vi "Oscilloscope_Interface.vi"() -> ()   [LabVIEW 2020]
uses:
  Tektronix 7000 Series/Library/Tektronix 7000 Series.lvlib
panel:
  out "Active_Channels":u16[](array[numeric])
  out "Get #Averages":i32
  in  "Go2":bool
  in  "Set Vertical Scale Button":bool
  in  "Channels Position":bool
  in  "Channels Bandwidth":bool
  in  "Default Setup Button":bool
  in  "Set Mode":bool
  in  "Autosetup":bool
  out "Oscilloscope Mode":string
  out "Synch Variable":bool
  out "S4":bool
  out "S3":bool
  out "S2":bool
  out "S1":bool
  out "Acquisition":bool
  in  "Configure Digital Channel":bool
  in  "Configure Measurement":bool
  in  "Configure Acquisition":bool
  in  "Timebase Configuration":bool
  in  "Cursor Configuration":bool
  in  "Histogram Configuration":bool
  in  "Set Horizontal Scale Button":bool
  in  "Go1":bool
  out "Measurement":dbl
  in  "Select a Channel for the Operation":i8(knob) scale=1.0..4.0
  in  "Trigger Configuration":bool
  in  "FunctionA":u16(ring) items=["Amplitude", "RMS", "Pk-Pk", "High", "Max", "Cycle RMS", "Low", "Min", "+Ovt shoot", "-Ovt shoot", "Cycle Mean", "Mean"]
  in  "Channels Configuration":bool
  out "Go!":bool
  out "Error!":bool
  in  "Synchronization":bool
  out "Display Message":string
  out "End Variable":bool
  out "Save Variable":bool
  in  "Operating Modes":bool
  in  "Pause Button":bool
  in  "Play Button":bool
  in  "End Button":bool
  in  "Guide Button":bool
  in  "Save Button":bool
  in  "Ch 4":bool
  in  "Ch 3":bool
  in  "Ch 2":bool
  in  "Ch 1":bool
  out "Running?":bool
  in  "Set Oscilloscope Mode":u16(ring) items=["Continuous", "Single"]
  in  "Set Sampling Mode":bool
  in  "Set Acquisition Mode":bool
  in  "Set Number of Averages":bool
  out "Master?":bool
  in  "Set Acquisition Mode":u16(ring) items=["Sample", "Peak Detect", "High resolution", "Average", "WFMDB", "Envelope"]
  out "Tektronix 7000 Oscilloscope":waveform(dbl)[](graph) caption="Oscilloscope"
  in  "Set Sampling Mode":u16(ring) items=["Real Time", "Equivalent Time", "Interpolation"]
  in  "Set #Averages":i32
  # "Tektronix DPO75002SX ATI Performance              Andrea Perna's Thesis"
  # "Channels Activation"
  # "Variables"
  # "Function"
  # "Set #Averages"
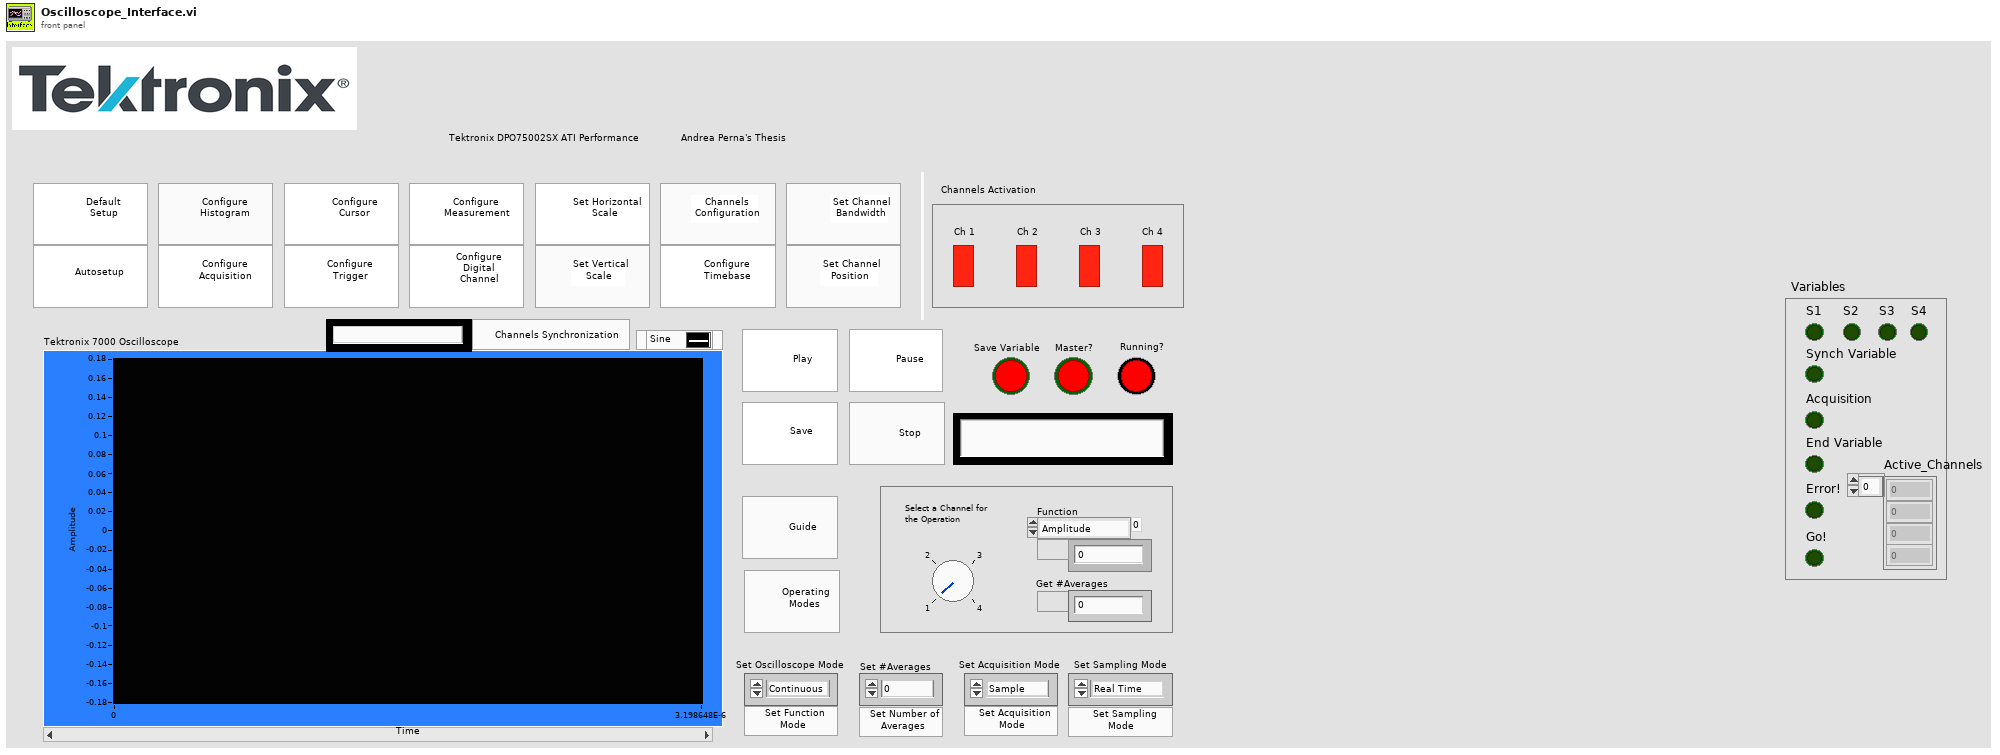
[diagram p1: front panel]
types:
  T1 = enum8{"Enabled", "Disabled", "Disabled and Grayed Out"}
  T2 = cluster{"Parameters(array)":string[], "Waveform Data":waveform(dbl)[], "array":u16[], bool}
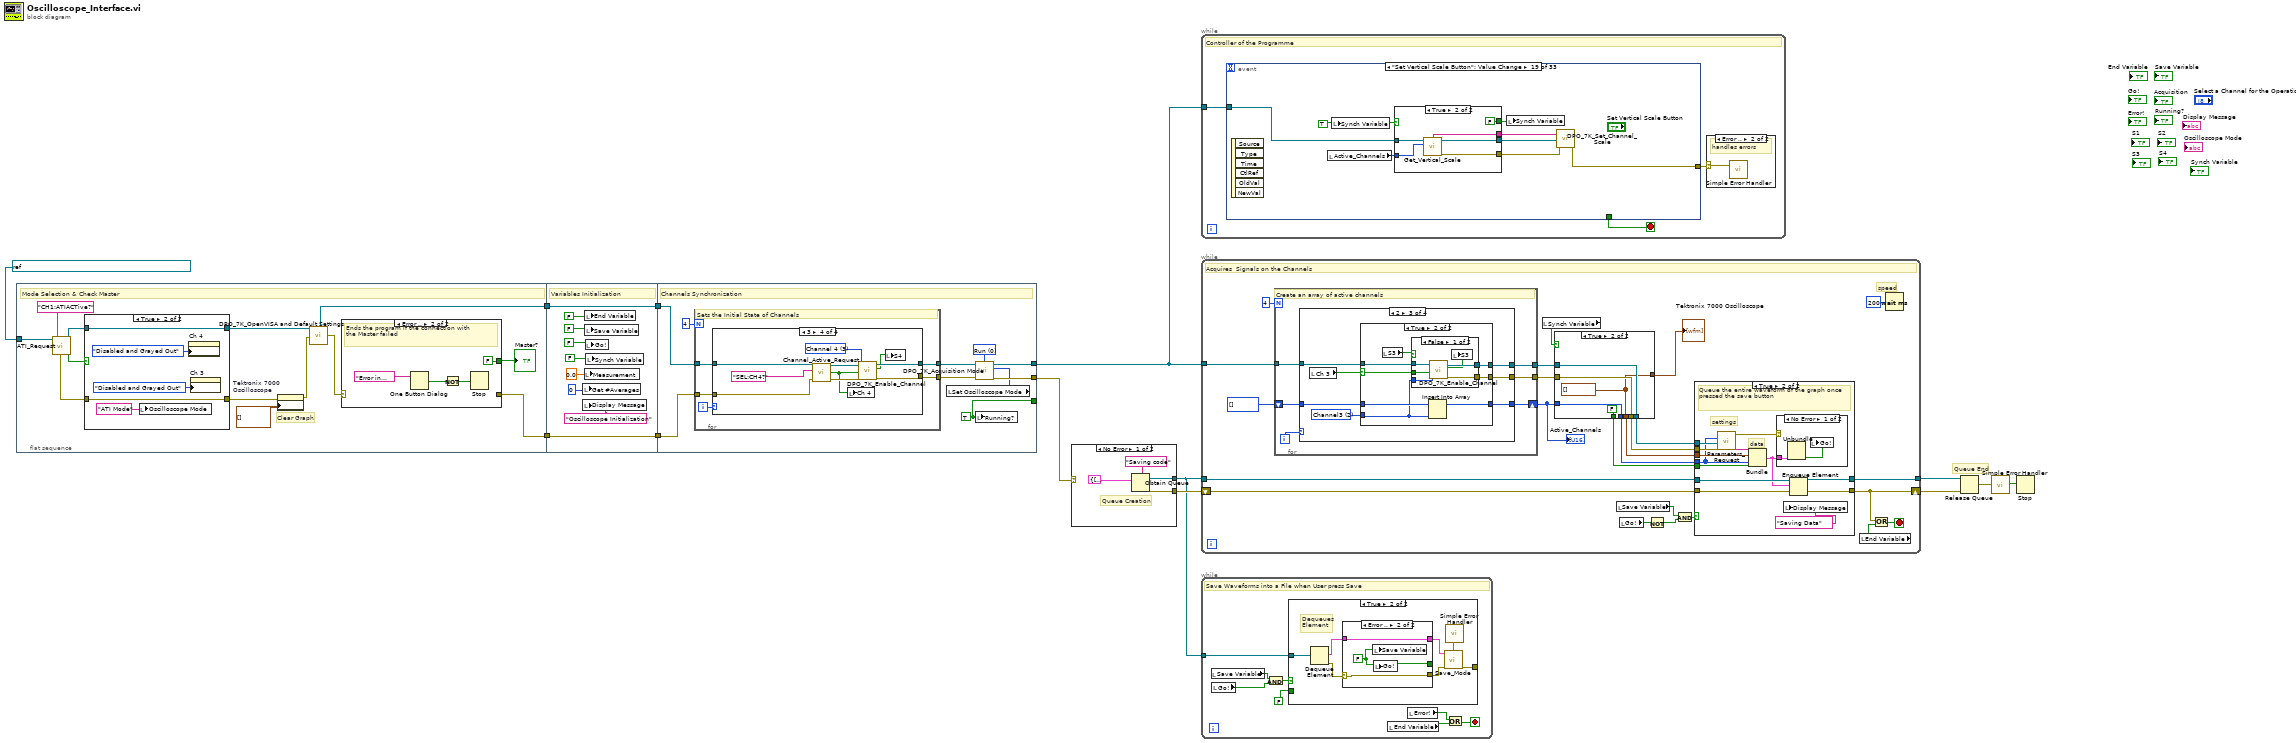
[diagram p0: block diagram]
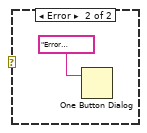
[diagram p2: hidden frame]
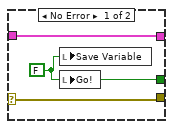
[diagram p4: hidden frame]
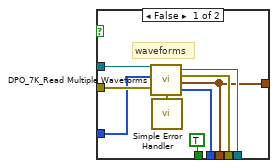
[diagram p5: hidden frame]
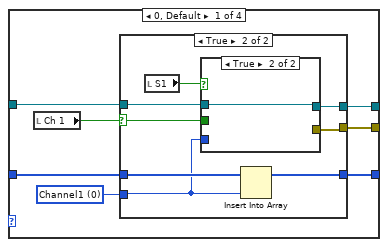
[diagram p6: hidden frame]
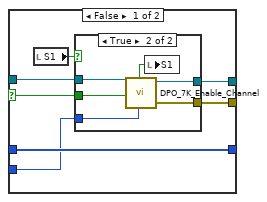
[diagram p7: hidden frame]
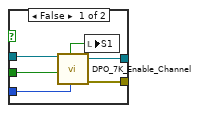
[diagram p9: hidden frame]
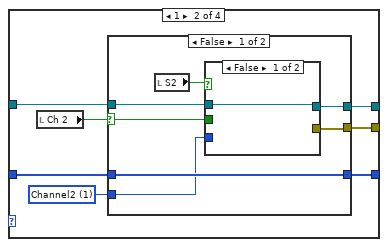
[diagram p10: hidden frame]
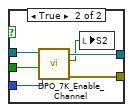
[diagram p11: hidden frame]
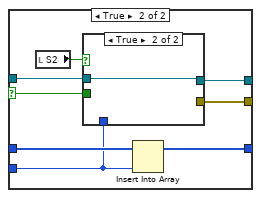
[diagram p12: hidden frame]
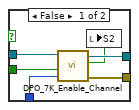
[diagram p13: hidden frame]
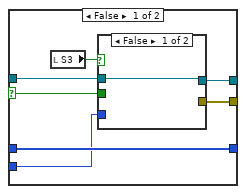
[diagram p14: hidden frame]
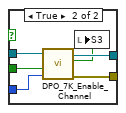
[diagram p15: hidden frame]
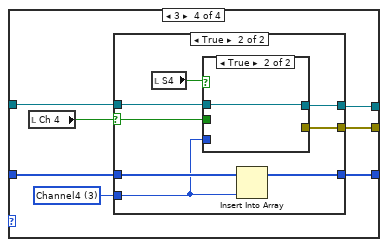
[diagram p17: hidden frame]
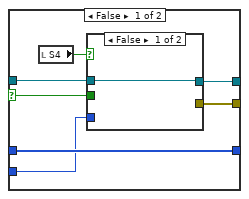
[diagram p18: hidden frame]
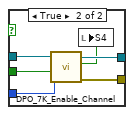
[diagram p19: hidden frame]
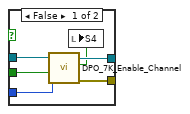
[diagram p20: hidden frame]
diagram:
  # "Queue End"
  n1 = flat-sequence {
    tunnel: [w15] -> w6
    tunnel: [w21] -> w4
    tunnel: refnum<visa-resource-name> "visa://10.16.3.95/TCPIP0::B300049-70KSX::inst0::INSTR" ("VISA resource name in") -> [w14]
    tunnel: w6 -> [w48]
    tunnel: [w48] -> w5
    tunnel: w4 -> [w43]
    tunnel: [w43] -> w3
    tunnel: w5 -> [w57]
    tunnel: [w51] -> w7
    tunnel: w3 -> [w56]
    tunnel: [w54] -> w2
    tunnel: [w49] -> _
    frame #0 {
      # "Clear Graph"
      # "Mode Selection & Check Master"
      n2 = call "ATI_Request.vi"("Command"="CH1:ATIACTive?", "VISA resource name"=w14) -> ("error out"=w17:errorcluster, "Active?"=w18:bool, "VISA resource name out"=w19:refnum<visa-resource-name>)  [unwired: 6 in, 1 out]
      n3 = case shown="True" w18 {
        tunnel: w19 -> [w28 w33]
        tunnel: w17 -> [w27 w32]
        tunnel: [w28 w33] -> w15
        tunnel: [w27 w32] -> w16
        frame False {
          n4 = local write "Oscilloscope Mode"("Tek Mode") -> ()
        }
        frame True {
          n5 = local write "Oscilloscope Mode"("ATI Mode") -> ()
          n6 = property on="Ch 4" class="Bool (strict)"("DisabledEnum"=T1."Disabled and Grayed Out" ("Disabled")) -> ()  [unwired: 2 in, 2 out]
          n7 = property on="Ch 3" class="Bool (strict)"("DisabledEnum"=T1."Disabled and Grayed Out" ("Disabled")) -> ()  [unwired: 2 in, 2 out]
        }
      }
      n8 = property on="Tektronix 7000 Oscilloscope" class="WFChart (strict)"(error in=w16, "History Data"=waveform(dbl)[][] []) -> (error out=w22:errorcluster)  [unwired: 1 in, 1 out]
      n9 = call "DPO_7K_OpenVISA and Default Settings.vi"("Error In"=w22, "VISA resource name in"=w15) -> ("error out"=w24:errorcluster)  [unwired: 8 in, 1 out]
      n10 = case shown="Error .." w24 {
        selector: w24 -> [w34 _]
        tunnel: [TRUE FALSE] -> w25
        tunnel: [w34 _] -> w21
        frame No Error {
          # "Ends the program if the connection with\nthe Master failed"
        }
        frame Error {
          # "Ends the program if the connection with\nthe Master failed"
          n11 = One Button Dialog(message="Error in communication with the master!") -> (true=w37:bool)  [unwired: 1 in]
          n12 = Not(x=w37) -> (.not. x?=w36:bool)
          n13 = Stop(stop? (T)=w36) -> ()
        }
      }
      "Master?" <- w25
    }
    frame #1 {
      # "Variables Initialization"
      n14 = local write "Get #Averages"(0) -> ()
      n15 = local write "Display Message"("Oscilloscope Initialization") -> ()
      n16 = local write "Measurement"(0.0) -> ()
      n17 = local write "End Variable"(FALSE ("End Variable")) -> ()
      n18 = local write "Save Variable"(FALSE ("Save Variable")) -> ()
      n19 = local write "Go!"(FALSE ("Vai!")) -> ()
      n20 = local write "Synch Variable"(FALSE ("Synch Variable")) -> ()
    }
    frame #2 {
      w49 = TRUE ("Running?")
      w52 = u16 0 items=["Run", "Stop"] ("Action")
      # "Channels Synchronization"
      n21 = for {
        N: 4 -> [_]
        tunnel: w57 -> [w62]
        tunnel: [w61] -> w55
        tunnel: w56 -> [w60]
        tunnel: [w59] -> w50
        i -> [w63]
        # "Sets the Initial State of Channels"
        n22 = case shown="3" w63 {
          tunnel: w62 -> [w72 w80 w90 w100]
          tunnel: [w69 w79 w89 w99] -> w59
          tunnel: [w66 w76 w86 w96] -> w61
          tunnel: w60 -> [w64 w74 w85 w94]
          frame 0, Default {
            w73 = u16 0 items=["Channel 1", "Channel 2", "Channel 3", "Channel 4", "Math 1", "Math 2", "Math 3", "Math 4", "Reference 1", "Reference 2", "Reference 3", "Reference 4"] ("Channel")
            n23 = call "Channel_Active_Request.vi"("error in (no error)"=w64, "Command"="SEL:CH1?", "VISA resource name"=w72) -> ("error out"=w70:errorcluster, "Active?"=w67:bool, "VISA resource name out"=w71:refnum<visa-resource-name>)  [unwired: 5 in, 1 out]
            n24 = local write "Ch 1"(w67) -> ()
            n25 = call "DPO_7K_Enable_Channel.vi"("Error In"=w70, "Activate?"=w67, "Channel"=w73, "VISA resource name in"=w71) -> ("Error Out"=w69:errorcluster, "State_Channel"=w65:bool, "VISA resource name out"=w66:refnum<visa-resource-name>)  [unwired: 5 in]
            n26 = local write "S1"(w65) -> ()
          }
          frame 1 {
            w83 = u16 1 items=["Channel 1", "Channel 2", "Channel 3", "Channel 4", "Math 1", "Math 2", "Math 3", "Math 4", "Reference 1", "Reference 2", "Reference 3", "Reference 4"] ("Channel")
            n27 = call "Channel_Active_Request.vi"("error in (no error)"=w74, "Command"="SEL:CH2?", "VISA resource name"=w80) -> ("error out"=w81:errorcluster, "Active?"=w77:bool, "VISA resource name out"=w82:refnum<visa-resource-name>)  [unwired: 5 in, 1 out]
            n28 = local write "Ch 2"(w77) -> ()
            n29 = call "DPO_7K_Enable_Channel.vi"("Error In"=w81, "Activate?"=w77, "Channel"=w83, "VISA resource name in"=w82) -> ("Error Out"=w79:errorcluster, "State_Channel"=w75:bool, "VISA resource name out"=w76:refnum<visa-resource-name>)  [unwired: 5 in]
            n30 = local write "S2"(w75) -> ()
          }
          frame 2 {
            w93 = u16 2 items=["Channel 1", "Channel 2", "Channel 3", "Channel 4", "Math 1", "Math 2", "Math 3", "Math 4", "Reference 1", "Reference 2", "Reference 3", "Reference 4"] ("Channel")
            n31 = call "Channel_Active_Request.vi"("error in (no error)"=w85, "Command"="SEL:CH3?", "VISA resource name"=w90) -> ("error out"=w91:errorcluster, "Active?"=w87:bool, "VISA resource name out"=w92:refnum<visa-resource-name>)  [unwired: 5 in, 1 out]
            n32 = local write "Ch 3"(w87) -> ()
            n33 = call "DPO_7K_Enable_Channel.vi"("Error In"=w91, "Activate?"=w87, "Channel"=w93, "VISA resource name in"=w92) -> ("Error Out"=w89:errorcluster, "State_Channel"=w84:bool, "VISA resource name out"=w86:refnum<visa-resource-name>)  [unwired: 5 in]
            n34 = local write "S3"(w84) -> ()
          }
          frame 3 {
            w103 = u16 3 items=["Channel 1", "Channel 2", "Channel 3", "Channel 4", "Math 1", "Math 2", "Math 3", "Math 4", "Reference 1", "Reference 2", "Reference 3", "Reference 4"] ("Channel")
            n35 = call "Channel_Active_Request.vi"("error in (no error)"=w94, "Command"="SEL:CH4?", "VISA resource name"=w100) -> ("error out"=w101:errorcluster, "Active?"=w97:bool, "VISA resource name out"=w102:refnum<visa-resource-name>)  [unwired: 5 in, 1 out]
            n36 = local write "Ch 4"(w97) -> ()
            n37 = call "DPO_7K_Enable_Channel.vi"("Error In"=w101, "Activate?"=w97, "Channel"=w103, "VISA resource name in"=w102) -> ("Error Out"=w99:errorcluster, "State_Channel"=w95:bool, "VISA resource name out"=w96:refnum<visa-resource-name>)  [unwired: 5 in]
            n38 = local write "S4"(w95) -> ()
          }
        }
      }
      n39 = local read "Set Oscilloscope Mode"() -> (w53:u16)
      n40 = call "DPO_7K_Acquisition Mode.vi"("Error In"=w50, "Mode"=w53, "Action"=w52, "VISA resource name in"=w55) -> ("Error Out"=w54:errorcluster, "VISA resource name out"=w51:refnum<visa-resource-name>)  [unwired: 6 in]
      n41 = local write "Running?"(w49) -> ()
    }
  }
  n42 = case shown="No Error" w2 {
    tunnel: [w107 _] -> w13
    tunnel: [w105 _] -> w12
    frame No Error {
      # "Queue Creation"
      n43 = Obtain Queue(name (unnamed)="Saving code", element data type=T2 {"Parameters(array)"=[], "Waveform Data"=[], "array"=[], FALSE} ("output cluster")) -> (queue out=w105:refnum<queue>, error out=w107:errorcluster)  [unwired: 3 in, 1 out]
    }
    frame Error {
      n44 = One Button Dialog(message="Error occurred during the initialization.") -> ()  [unwired: 1 in, 1 out]
    }
  }
  n45 = while {
    tunnel: w12 -> [w116]
    stop <- w114 stop-if-true
    # "Save Waveforms into a File when User press Save"
    n46 = local read "Save Variable"() -> (w111:bool)
    n47 = local read "Go!"() -> (w110:bool)
    n48 = And(x=w111, y=w110) -> (x .and. y?=w112:bool)
    n49 = case shown="True" w112 {
      tunnel: w116 -> [_ w122]
      tunnel: FALSE -> [_ _]
      tunnel: [_ w117] -> _
      frame False {
      }
      frame True {
        # "Dequeues\nElement"
        n50 = Dequeue Element(queue=w122) -> (element=w119:T2, error out=w121:errorcluster)  [unwired: 2 in, 2 out]
        n51 = case shown="Error .." w121 {
          selector: w121 -> [w125 w127]
          tunnel: [w125 w127] -> w120
          tunnel: w119 -> [w124 w128]
          tunnel: [w124 w128] -> w118
          tunnel: [w123 w126] -> _
          frame No Error {
            w123 = FALSE
            n52 = local write "Save Variable"(w123) -> ()
            n53 = local write "Go!"(w123) -> ()
          }
          frame Error {
            w126 = FALSE
            n54 = local write "Save Variable"(w126) -> ()
            n55 = local write "Go!"(w126) -> ()
          }
        }
        n56 = call "Save_Mode.vi"("error in (no error)"=w120, "Data"=w118) -> ("error out"=w117:errorcluster)  [unwired: 7 in]
        n57 = call <vilib>:"Simple Error Handler.vi"("error in (no error)"=w117) -> ()  [unwired: 4 in, 5 out]
      }
    }
    n58 = local read "End Variable"() -> (w115:bool)
    n59 = local read "Error!"() -> (w113:bool)
    n60 = Or(x=w113, y=w115) -> (x .or. y?=w114:bool)
  }
  n61 = while {
    tunnel: w7 -> [w130]
    stop <- w131 stop-if-true
    # "Controller of the Programme"
    n62 = event shown="[18] \"Set Vertical Scale Button\": Value Change" {
      selector: _ -> [_ _ _ _ _ _ _ _ _ _ _ _ _ _ _ _ _ _ _ _ _ _ _ _ _ _ _ _ _ _ _ _ _]
      dyn-events: _ -> [_ _ _ _ _ _ _ _ _ _ _ _ _ _ _ _ _ _ _ _ _ _ _ _ _ _ _ _ _ _ _ _ _]
      timeout: _ -> [_ _ _ _ _ _ _ _ _ _ _ _ _ _ _ _ _ _ _ _ _ _ _ _ _ _ _ _ _ _ _ _ _]
      tunnel: [_ _ _ _ _ _ _ _ _ _ _ _ _ _ _ w202 _ _ _ _ _ _ _ _ _ _ _ _ _ w315 _ _ _] -> w131
      tunnel: w130 -> [w134 w136 w138 w140 w142 w144 w148 w154 w157 w159 w162 w163 _ w172 _ w201 w270 w272 w278 w289 w298 _ _ _ _ _ w302 _ w308 _ w326 w467 w472]
      tunnel: [w133 w135 w137 w139 w141 w143 w147 w153 w156 w158 w160 w164 _ w171 _ w199 w269 w271 w280 w288 w297 _ _ _ _ _ w299 _ w307 _ w325 w466 w471] -> w129
      event "Set Horizontal Scale Button": Value Change {
        n63 = event-data() -> ()  [unwired: 1 in, 6 out]
        n64 = call "DPO_7K_Set_Horizontal_Scale.vi"("VISA resource name in"=w134) -> ("Error Out"=w133:errorcluster)  [unwired: 9 in, 1 out]
      }
      event "Histogram Configuration": Value Change {
        n65 = event-data() -> ()  [unwired: 1 in, 6 out]
        n66 = call "Configure Histogram.vi"("VISA resource name"=w136) -> ("error out"=w135:errorcluster)  [unwired: 13 in, 1 out]
      }
      event "Cursor Configuration": Value Change {
        n67 = event-data() -> ()  [unwired: 1 in, 6 out]
        n68 = call "Configure Cursors.vi"("VISA resource name"=w138) -> ("error out"=w137:errorcluster)  [unwired: 13 in, 1 out]
      }
      event "Timebase Configuration": Value Change {
        n69 = event-data() -> ()  [unwired: 1 in, 6 out]
        n70 = call "Configure Timebase.vi"("VISA resource name"=w140) -> ("error out"=w139:errorcluster)  [unwired: 9 in, 1 out]
      }
      event "Configure Measurement": Value Change {
        n71 = event-data() -> ()  [unwired: 1 in, 6 out]
        n72 = call "Configure Measurement.vi"("VISA resource name"=w142) -> ("error out"=w141:errorcluster)  [unwired: 13 in, 1 out]
      }
      event "Configure Acquisition": Value Change {
        n73 = event-data() -> ()  [unwired: 1 in, 6 out]
        n74 = call "Configure Acquisition.vi"("VISA resource name"=w144) -> ("error out"=w143:errorcluster)  [unwired: 13 in, 1 out]
      }
      event "Go2": Value Change {
        w145 = TRUE ("Synch Variable")
        n75 = event-data() -> ()  [unwired: 1 in, 6 out]
        n76 = local write "Synch Variable"(w145) -> ()
        n77 = case shown="True" w145 {
          tunnel: w148 -> [w152 _]
          tunnel: [w151 _] -> w147
          tunnel: [FALSE _] -> w146
          frame True {
            n78 = call "Get_Averages.vi"("VISA resource name"=w152) -> ("error out"=w151:errorcluster, "number"=→"Get #Averages":i32)  [unwired: 7 in, 2 out]
          }
          frame False {
          }
        }
        n79 = local write "Synch Variable"(w146) -> ()
      }
      event "Configure Digital Channel": Value Change {
        n80 = event-data() -> ()  [unwired: 1 in, 6 out]
        n81 = call "Configure Digital Channel.vi"("VISA resource name"=w154) -> ("error out"=w153:errorcluster)  [unwired: 9 in, 1 out]
      }
      event "Set Sampling Mode": Value Change {
        n82 = event-data() -> ()  [unwired: 1 in, 6 out]
        n83 = call "DPO_7K_Set_Sampling_Mode.vi"("Sampling Mode"="Set Sampling Mode", "VISA resource name in"=w157) -> ("Error Out"=w156:errorcluster)  [unwired: 8 in, 1 out]
      }
      event "Trigger Configuration": Value Change {
        n84 = event-data() -> ()  [unwired: 1 in, 6 out]
        n85 = call "DPO_7K_Set_Edge_Trigger.vi"("VISA resource name in"=w159) -> ("Error Out"=w158:errorcluster)  [unwired: 9 in, 1 out]
      }
      event "Set Acquisition Mode": Value Change {
        n86 = event-data() -> ()  [unwired: 1 in, 6 out]
        n87 = call "DPO_7K_Set_Acquisition_Mode.vi"("Acquisition Mode"="Set Acquisition Mode", "VISA resource name in"=w162) -> ("Error Out"=w160:errorcluster)  [unwired: 8 in, 1 out]
      }
      event "Channels Configuration": Value Change {
        n88 = event-data() -> ()  [unwired: 1 in, 6 out]
        n89 = call "Configure Channel.vi"("VISA resource name"=w163) -> ("error out"=w164:errorcluster)  [unwired: 13 in, 1 out]
      }
      event "Operating Modes": Value Change {
        n90 = event-data() -> ()  [unwired: 1 in, 6 out]
        n91 = call "Initial_Menu.vi"() -> ()  [unwired: 12 in]
      }
      event "Go1": Value Change {
        w170 = TRUE
        n92 = event-data() -> ()  [unwired: 1 in, 6 out]
        n93 = local read "Select a Channel for the Operation"() -> (w169:i8)
        n94 = case shown="1, Default" w169 {
          tunnel: [w174 w176 w178 w180] -> w168
          tunnel: [w173 w175 w177 w179] -> w167
          frame 1, Default {
            w174 = u16 0 items=["Channel1", "Channel2", "Channel3", "Channel4", "Math1", "Math2", "Math3", "Math3", "Reference1", "Reference2", "Reference3", "Reference4"] ("Channel (0:Channel1)")
            n95 = local read "Ch 1"() -> (w173:bool)
          }
          frame 2 {
            w176 = u16 1 items=["Channel1", "Channel2", "Channel3", "Channel4", "Math1", "Math2", "Math3", "Math3", "Reference1", "Reference2", "Reference3", "Reference4"] ("Channel (0:Channel1)")
            n96 = local read "Ch 2"() -> (w175:bool)
          }
          frame 3 {
            w178 = u16 2 items=["Channel1", "Channel2", "Channel3", "Channel4", "Math1", "Math2", "Math3", "Math3", "Reference1", "Reference2", "Reference3", "Reference4"] ("Channel (0:Channel1)")
            n97 = local read "Ch 3"() -> (w177:bool)
          }
          frame 4 {
            w180 = u16 3 items=["Channel1", "Channel2", "Channel3", "Channel4", "Math1", "Math2", "Math3", "Math3", "Reference1", "Reference2", "Reference3", "Reference4"] ("Channel (0:Channel1)")
            n98 = local read "Ch 4"() -> (w179:bool)
          }
        }
        n99 = local write "Synch Variable"(w170) -> ()
        n100 = Equal?(x=TRUE, y=w167) -> (x = y?=w165:bool)
        n101 = case shown="True" w165 {
          selector: w165 -> [w181 _]
          tunnel: w172 -> [_ w188]
          tunnel: [_ w187] -> w171
          tunnel: w170 -> [_ _]
          tunnel: w168 -> [_ w185]
          frame False {
            n102 = local write "Synch Variable"(w181) -> ()
            n103 = One Button Dialog(message="The selected channel is not active.") -> (true=w182:bool)  [unwired: 1 in]
            n104 = Not(x=w182) -> ()  [unwired: 1 out]
          }
          frame True {
            n105 = call "Read Waveform Measurement (Amplitude).vi"("VISA resource name"=w188, "Maximum Time (25000ms)"=u32 25000, "Channel (0:Channel1)"=w185, "Function (0:Amplitude)"="FunctionA") -> ("Measurement"=→"Measurement":dbl, "Finish"=w184:bool, "error out"=w187:errorcluster)  [unwired: 8 in, 1 out]
            n106 = local write "Synch Variable"(w184) -> ()
          }
        }
      }
      event Panel Close? {
        n107 = event-data() -> ()  [unwired: 1 in, 4 out]
        n108 = Two Button Dialog(message="Do you want to quit the programme?", 1:"No" ("F button name (\"Cancel\")"), 2:"Yes" ("T button name (\"OK\")")) -> (T button?=w192:bool)
        n109 = case shown="False" w192 {
          tunnel: [FALSE TRUE] -> w191
          frame False {
          }
          frame True {
          }
        }
        n110 = Not(x=w192) -> (.not. x?=w193:bool)
        n111 = local write "End Variable"(w191) -> ()
        n112 = event-data("Discard?"=w193) -> ()  [unwired: 1 in, 1 out]
      }
      event Menu Selection (User) {
        # "Handle the Real Time Menu"
        n113 = event-data() -> ("ItemTag"=w200:string)  [unwired: 1 in]
        n114 = case shown="\"Default Setup\"" w200 {
          tunnel: [_ _ _ _ _ _ _ _ _ _ _ _ _ _ w233 _ _ _ _ _ _ _ _ _] -> w202
          tunnel: w201 -> [w203 w206 w208 w210 _ w215 _ w218 w219 w224 w227 _ w229 w231 _ w239 w241 w243 w245 w247 w250 w251 w258 w262]
          tunnel: [w204 w205 w207 w209 _ w214 _ w217 w220 w223 w226 _ w228 w230 _ w240 w242 w244 w246 w248 w249 w252 w253 w261] -> w199
          frame "Set Channel Scale" {
            n115 = call "DPO_7K_Set_Channel_Scale.vi"("VISA resource name in"=w203) -> ("Error Out"=w204:errorcluster)  [unwired: 9 in, 1 out]
          }
          frame "Set Channel Position" {
            n116 = call "DPO_7K_Set_Channel_Position.vi"("VISA resource name in"=w206) -> ("Error Out"=w205:errorcluster)  [unwired: 9 in, 1 out]
          }
          frame "Set Channel Bandwidth" {
            n117 = call "DPO_7K_Set_Channel_Bandwidth.vi"("VISA resource name in"=w208) -> ("Error Out"=w207:errorcluster)  [unwired: 9 in, 1 out]
          }
          frame "Channels Configuration" {
            n118 = call "Configure Channel.vi"("VISA resource name"=w210) -> ("error out"=w209:errorcluster)  [unwired: 13 in, 1 out]
          }
          frame "Operating Modes" {
            n119 = call "Initial_Menu.vi"() -> ()  [unwired: 12 in]
          }
          frame "Run" {
            w213 = u16 0 items=["Run", "Stop"] ("Action")
            n120 = local read "Set Oscilloscope Mode"() -> (w212:u16)
            n121 = call "DPO_7K_Acquisition Mode.vi"("Mode"=w212, "Action"=w213, "VISA resource name in"=w215) -> ("Error Out"=w214:errorcluster)  [unwired: 7 in, 1 out]
            n122 = local write "Running?"(TRUE ("Running?")) -> ()
          }
          frame "Save Waveform" {
            n123 = local write "Save Variable"(TRUE ("Save Variable")) -> ()
          }
          frame "Max Value Measurement" {
            n124 = call "DPO_7K_MaxValue_measurement.vi"("VISA resource name in"=w218) -> ("Error Out"=w217:errorcluster)  [unwired: 8 in, 2 out]
          }
          frame "Min Value Measurement" {
            n125 = call "DPO_7K_MinValue_measurement.vi"("VISA resource name in"=w219) -> ("Error Out"=w220:errorcluster)  [unwired: 8 in, 2 out]
          }
          frame "Pause" {
            w225 = u16 1 items=["Run", "Stop"] ("Action")
            n126 = local read "Set Oscilloscope Mode"() -> (w222:u16)
            n127 = call "DPO_7K_Acquisition Mode.vi"("Mode"=w222, "Action"=w225, "VISA resource name in"=w224) -> ("Error Out"=w223:errorcluster)  [unwired: 7 in, 1 out]
            n128 = local write "Running?"(FALSE ("Running?")) -> ()
          }
          frame "Horizontal Scale", Default {
            n129 = call "DPO_7K_Set_Horizontal_Scale.vi"("VISA resource name in"=w227) -> ("Error Out"=w226:errorcluster)  [unwired: 9 in, 1 out]
          }
          frame "Oscilloscope Guide" {
            n130 = call "Oscilloscope_Info_Guide.vi"() -> ()  [unwired: 12 in]
          }
          frame "Channel Position" {
            n131 = call "DPO_7K_Get_Channel_Position.vi"("VISA resource name in"=w229) -> ("Error Out"=w228:errorcluster)  [unwired: 8 in, 2 out]
          }
          frame "Channel Scale" {
            n132 = call "DPO_7K_Get_Channel_Scale.vi"("VISA resource name in"=w231) -> ("Error Out"=w230:errorcluster)  [unwired: 8 in, 2 out]
          }
          frame "End Programme" {
            n133 = Two Button Dialog(message="Do you want to end the programme?", 1:"No" ("F button name (\"Cancel\")"), 2:"Yes" ("T button name (\"OK\")")) -> (T button?=w233:bool)
            n134 = case shown="False" w233 {
              tunnel: [FALSE TRUE] -> w232
              frame False {
              }
              frame True {
              }
            }
            n135 = local write "End Variable"(w232) -> ()
          }
          frame "Trigger" {
            n136 = call "DPO_7K_Set_Edge_Trigger.vi"("VISA resource name in"=w239) -> ("Error Out"=w240:errorcluster)  [unwired: 9 in, 1 out]
          }
          frame "Cursor" {
            n137 = call "Configure Cursors.vi"("VISA resource name"=w241) -> ("error out"=w242:errorcluster)  [unwired: 13 in, 1 out]
          }
          frame "Histogram" {
            n138 = call "Configure Histogram.vi"("VISA resource name"=w243) -> ("error out"=w244:errorcluster)  [unwired: 13 in, 1 out]
          }
          frame "Measurement" {
            n139 = call "Configure Measurement.vi"("VISA resource name"=w245) -> ("error out"=w246:errorcluster)  [unwired: 13 in, 1 out]
          }
          frame "Digital Channel" {
            n140 = call "Configure Digital Channel.vi"("VISA resource name"=w247) -> ("error out"=w248:errorcluster)  [unwired: 9 in, 1 out]
          }
          frame "Acquisition" {
            n141 = call "Configure Acquisition.vi"("VISA resource name"=w250) -> ("error out"=w249:errorcluster)  [unwired: 13 in, 1 out]
          }
          frame "Timebase" {
            n142 = call "Configure Timebase.vi"("VISA resource name"=w251) -> ("error out"=w252:errorcluster)  [unwired: 9 in, 1 out]
          }
          frame "Default Setup" {
            n143 = Two Button Dialog(message="Do you really want to set the settings to default?", 1:"No" ("F button name (\"Cancel\")"), 2:"Yes" ("T button name (\"OK\")")) -> (T button?=w254:bool)
            n144 = case shown="True" w254 {
              tunnel: w258 -> [_ w260]
              tunnel: [_ w259] -> w253
              frame False {
              }
              frame True {
                n145 = call "DPO_7k_Default_Setup.vi"("VISA resource name in"=w260) -> ("Error out"=w259:errorcluster)  [unwired: 9 in, 1 out]
              }
            }
          }
          frame "Autosetup" {
            n146 = Two Button Dialog(message="Do you really want to do the autosetup?", 1:"No" ("F button name (\"Cancel\")"), 2:"Yes" ("T button name (\"OK\")")) -> (T button?=w263:bool)
            n147 = case shown="True" w263 {
              tunnel: w262 -> [_ w268]
              tunnel: [_ w267] -> w261
              frame False {
              }
              frame True {
                n148 = call "Autosetup.vi"("VISA resource name"=w268) -> ("error out"=w267:errorcluster)  [unwired: 9 in, 1 out]
              }
            }
          }
        }
      }
      event "Channels Bandwidth": Value Change {
        n149 = event-data() -> ()  [unwired: 1 in, 6 out]
        n150 = call "DPO_7K_Set_Channel_Bandwidth.vi"("VISA resource name in"=w270) -> ("Error Out"=w269:errorcluster)  [unwired: 9 in, 1 out]
      }
      event "Channels Position": Value Change {
        n151 = event-data() -> ()  [unwired: 1 in, 6 out]
        n152 = call "DPO_7K_Set_Channel_Position.vi"("VISA resource name in"=w272) -> ("Error Out"=w271:errorcluster)  [unwired: 9 in, 1 out]
      }
      event "Set Vertical Scale Button": Value Change {
        w279 = TRUE ("Synch Variable")
        n153 = event-data() -> ()  [unwired: 1 in, 6 out]
        n154 = local read "Active_Channels"() -> (w274:u16[])
        n155 = local write "Synch Variable"(w279) -> ()
        n156 = case shown="True" w279 {
          tunnel: w278 -> [w281 w287]
          tunnel: [_ w286] -> w277
          tunnel: [w281 w285] -> w276
          tunnel: [_ w284] -> w275
          tunnel: w274 -> [_ w283]
          tunnel: [_ FALSE] -> w273
          frame False {
          }
          frame True {
            n157 = call "Get_Vertical_Scale.vi"("Active_Channels"=w283, "VISA resource name"=w287) -> ("error out"=w286:errorcluster, "Vertical_Parameters"=w284:string[], "VISA resource name out"=w285:refnum<visa-resource-name>)  [unwired: 6 in]
          }
        }
        n158 = local write "Synch Variable"(w273) -> ()
        n159 = call "DPO_7K_Set_Channel_Scale.vi"("Vertical_Parameters"=w275, "Error In"=w277, "VISA resource name in"=w276) -> ("Error Out"=w280:errorcluster)  [unwired: 7 in, 1 out]
      }
      event "Autosetup": Value Change {
        n160 = event-data() -> ()  [unwired: 1 in, 6 out]
        n161 = Two Button Dialog(message="Do you really want to do the autosetup?", 1:"No" ("F button name (\"Cancel\")"), 2:"Yes" ("T button name (\"OK\")")) -> (T button?=w290:bool)
        n162 = case shown="True" w290 {
          tunnel: w289 -> [_ w295]
          tunnel: [_ w294] -> w288
          frame False {
          }
          frame True {
            n163 = call "Autosetup.vi"("VISA resource name"=w295) -> ("error out"=w294:errorcluster)  [unwired: 9 in, 1 out]
          }
        }
      }
      event "Set Number of Averages": Value Change {
        # "da sistemare per stampare il valore di medie ad\ninizio programma ed in questo andare ad aggiornare il valore"
        n164 = event-data() -> ()  [unwired: 1 in, 6 out]
        n165 = call "DPO_7K_Set_Number_of_Averages.vi"("Number of Waveforms"="Set #Averages", "VISA resource name in"=w298) -> ("Error Out"=w297:errorcluster)  [unwired: 8 in, 1 out]
      }
      event "Ch 1": Value Change {
        n166 = event-data() -> ()  [unwired: 1 in, 6 out]
      }
      event "Ch 2": Value Change {
        n167 = event-data() -> ()  [unwired: 1 in, 6 out]
      }
      event "Ch 3": Value Change {
        n168 = event-data() -> ()  [unwired: 1 in, 6 out]
      }
      event "Ch 4": Value Change {
        # "Handles All Events Of The Programme"
        n169 = event-data() -> ()  [unwired: 1 in, 6 out]
      }
      event "Guide Button": Value Change {
        n170 = event-data() -> ()  [unwired: 1 in, 6 out]
        n171 = call "Oscilloscope_Info_Guide.vi"() -> ()  [unwired: 12 in]
      }
      event "Set Mode": Value Change {
        n172 = event-data() -> ()  [unwired: 1 in, 6 out]
        n173 = local read "Running?"() -> (w303:bool)
        n174 = case shown="False" w303 {
          tunnel: [w304 w305] -> w301
          frame False {
            w304 = u16 1 items=["Run", "Stop"] ("Action")
          }
          frame True {
            w305 = u16 0 items=["Run", "Stop"] ("Action")
          }
        }
        n175 = call "DPO_7K_Acquisition Mode.vi"("Mode"="Set Oscilloscope Mode", "Action"=w301, "VISA resource name in"=w302) -> ("Error Out"=w299:errorcluster)  [unwired: 7 in, 1 out]
      }
      event "Save Button": Value Change {
        n176 = event-data() -> ()  [unwired: 1 in, 6 out]
        n177 = local write "Save Variable"(TRUE ("Save Variable")) -> ()
      }
      event "Default Setup Button": Value Change {
        # "Resets the instrument to factory default settings"
        n178 = event-data() -> ()  [unwired: 1 in, 6 out]
        n179 = Two Button Dialog(message="Do you really want to set settings to the default values?", 1:"No" ("F button name (\"Cancel\")"), 2:"Yes" ("T button name (\"OK\")")) -> (T button?=w309:bool)
        n180 = case shown="True" w309 {
          tunnel: w308 -> [_ w314]
          tunnel: [_ w313] -> w307
          frame False {
          }
          frame True {
            n181 = call "DPO_7k_Default_Setup.vi"("VISA resource name in"=w314) -> ("Error out"=w313:errorcluster)  [unwired: 9 in, 1 out]
          }
        }
      }
      event "End Button": Value Change {
        n182 = event-data() -> ()  [unwired: 1 in, 6 out]
        n183 = Two Button Dialog(message="Do you want to end the programme?", 1:"No" ("F button name (\"Cancel\")"), 2:"Yes" ("T button name (\"OK\")")) -> (T button?=w315:bool)
        n184 = case shown="False" w315 {
          tunnel: [FALSE ("End Variable") TRUE ("End Variable")] -> w316
          frame False {
          }
          frame True {
          }
        }
        n185 = local write "End Variable"(w316) -> ()
      }
      event "Synchronization": Value Change {
        w324 = TRUE ("Synch Variable")
        n186 = event-data() -> ()  [unwired: 1 in, 6 out]
        n187 = local write "Display Message"("Synchronization") -> ()
        n188 = local write "Synch Variable"(w324) -> ()
        n189 = for {
          N: 4 -> [_]
          tunnel: [w330] -> w325
          tunnel: w326 -> [w329]
          tunnel: w324 -> [_]
          tunnel: [FALSE] -> w323
          i -> [w331]
          # "Synchronize Channels"
          n190 = case shown="3" w331 {
            tunnel: [w335 w368 w401 w435] -> w330
            tunnel: w329 -> [w333 w367 w400 w433]
            frame 0, Default {
              w338 = u16 0 items=["Channel 1", "Channel 2", "Channel 3", "Channel 4", "Math 1", "Math 2", "Math 3", "Math 4", "Reference 1", "Reference 2", "Reference 3", "Reference 4"] ("Channel")
              n191 = call "Channel_Active_Request.vi"("Command"="SEL:CH1?", "VISA resource name"=w333) -> ("error out"=w334:errorcluster, "Active?"=w332:bool, "VISA resource name out"=w336:refnum<visa-resource-name>)  [unwired: 6 in, 1 out]
              n192 = case shown="False" w332 {
                selector: w332 -> [w339 w353]
                tunnel: w338 -> [w344 w357]
                tunnel: w336 -> [w342 w356]
                tunnel: [w340 w355] -> w335
                tunnel: w334 -> [w341 w354]
                frame False {
                  n193 = local read "Ch 1"() -> (w343:bool)
                  n194 = case shown="True" w343 {
                    tunnel: w344 -> [_ w351]
                    tunnel: w342 -> [_ w350]
                    tunnel: w341 -> [w345 w348]
                    tunnel: [w345 w347] -> w340
                    tunnel: w339 -> [_ w346]
                    frame False {
                    }
                    frame True {
                      n195 = call "DPO_7K_Enable_Channel.vi"("Error In"=w348, "Activate?"=w346, "Channel"=w351, "VISA resource name in"=w350) -> ("Error Out"=w347:errorcluster, "State_Channel"=w349:bool)  [unwired: 5 in, 1 out]
                      n196 = local write "Ch 1"(w349) -> ()
                      n197 = local write "S1"(w349) -> ()
                    }
                  }
                }
                frame True {
                  n198 = local read "Ch 1"() -> (w352:bool)
                  n199 = case shown="False" w352 {
                    tunnel: w357 -> [w363 _]
                    tunnel: w356 -> [w362 _]
                    tunnel: [w361 w364] -> w355
                    tunnel: w354 -> [w360 w364]
                    tunnel: w353 -> [w359 _]
                    frame False {
                      n200 = call "DPO_7K_Enable_Channel.vi"("Error In"=w360, "Activate?"=w359, "Channel"=w363, "VISA resource name in"=w362) -> ("Error Out"=w361:errorcluster, "State_Channel"=w358:bool)  [unwired: 5 in, 1 out]
                      n201 = local write "Ch 1"(w358) -> ()
                      n202 = local write "S1"(w358) -> ()
                    }
                    frame True {
                    }
                  }
                }
              }
            }
            frame 1 {
              w366 = u16 1 items=["Channel 1", "Channel 2", "Channel 3", "Channel 4", "Math 1", "Math 2", "Math 3", "Math 4", "Reference 1", "Reference 2", "Reference 3", "Reference 4"] ("Channel")
              n203 = call "Channel_Active_Request.vi"("Command"="SEL:CH2?", "VISA resource name"=w367) -> ("error out"=w369:errorcluster, "Active?"=w365:bool, "VISA resource name out"=w370:refnum<visa-resource-name>)  [unwired: 6 in, 1 out]
              n204 = case shown="True" w365 {
                selector: w365 -> [w372 w386]
                tunnel: w370 -> [w375 w390]
                tunnel: w369 -> [w374 w389]
                tunnel: [w373 w388] -> w368
                tunnel: w366 -> [w377 w387]
                frame False {
                  n205 = local read "Ch 2"() -> (w376:bool)
                  n206 = case shown="False" w376 {
                    tunnel: w377 -> [_ w379]
                    tunnel: w375 -> [_ w381]
                    tunnel: w374 -> [w378 w384]
                    tunnel: [w378 w383] -> w373
                    tunnel: w372 -> [_ w380]
                    frame False {
                    }
                    frame True {
                      n207 = call "DPO_7K_Enable_Channel.vi"("Error In"=w384, "Activate?"=w380, "Channel"=w379, "VISA resource name in"=w381) -> ("Error Out"=w383:errorcluster, "State_Channel"=w382:bool)  [unwired: 5 in, 1 out]
                      n208 = local write "Ch 2"(w382) -> ()
                      n209 = local write "S2"(w382) -> ()
                    }
                  }
                }
                frame True {
                  n210 = local read "Ch 2"() -> (w385:bool)
                  n211 = case shown="False" w385 {
                    tunnel: w390 -> [w396 _]
                    tunnel: w389 -> [w395 w397]
                    tunnel: w386 -> [w394 _]
                    tunnel: [w393 w397] -> w388
                    tunnel: w387 -> [w392 _]
                    frame False {
                      n212 = call "DPO_7K_Enable_Channel.vi"("Error In"=w395, "Activate?"=w394, "Channel"=w392, "VISA resource name in"=w396) -> ("Error Out"=w393:errorcluster, "State_Channel"=w391:bool)  [unwired: 5 in, 1 out]
                      n213 = local write "S2"(w391) -> ()
                      n214 = local write "Ch 2"(w391) -> ()
                    }
                    frame True {
                    }
                  }
                }
              }
            }
            frame 2 {
              w399 = u16 2 items=["Channel 1", "Channel 2", "Channel 3", "Channel 4", "Math 1", "Math 2", "Math 3", "Math 4", "Reference 1", "Reference 2", "Reference 3", "Reference 4"] ("Channel")
              n215 = call "Channel_Active_Request.vi"("Command"="SEL:CH3?", "VISA resource name"=w400) -> ("error out"=w402:errorcluster, "Active?"=w398:bool, "VISA resource name out"=w403:refnum<visa-resource-name>)  [unwired: 6 in, 1 out]
              n216 = case shown="True" w398 {
                selector: w398 -> [w407 w418]
                tunnel: w403 -> [w405 w423]
                tunnel: w402 -> [w408 w422]
                tunnel: [w409 w421] -> w401
                tunnel: w399 -> [w410 w420]
                frame False {
                  n217 = local read "Ch 3"() -> (w406:bool)
                  n218 = case shown="True" w406 {
                    tunnel: w410 -> [_ w414]
                    tunnel: [w411 w417] -> w409
                    tunnel: w408 -> [w411 w416]
                    tunnel: w407 -> [_ w415]
                    tunnel: w405 -> [_ w413]
                    frame False {
                    }
                    frame True {
                      n219 = call "DPO_7K_Enable_Channel.vi"("Error In"=w416, "Activate?"=w415, "Channel"=w414, "VISA resource name in"=w413) -> ("Error Out"=w417:errorcluster, "State_Channel"=w412:bool)  [unwired: 5 in, 1 out]
                      n220 = local write "Ch 3"(w412) -> ()
                      n221 = local write "S3"(w412) -> ()
                    }
                  }
                }
                frame True {
                  n222 = local read "Ch 3"() -> (w419:bool)
                  n223 = case shown="False" w419 {
                    tunnel: w423 -> [w429 _]
                    tunnel: w422 -> [w428 w430]
                    tunnel: [w427 w430] -> w421
                    tunnel: w420 -> [w426 _]
                    tunnel: w418 -> [w424 _]
                    frame False {
                      n224 = call "DPO_7K_Enable_Channel.vi"("Error In"=w428, "Activate?"=w424, "Channel"=w426, "VISA resource name in"=w429) -> ("Error Out"=w427:errorcluster, "State_Channel"=w425:bool)  [unwired: 5 in, 1 out]
                      n225 = local write "Ch 3"(w425) -> ()
                      n226 = local write "S3"(w425) -> ()
                    }
                    frame True {
                    }
                  }
                }
              }
            }
            frame 3 {
              w431 = u16 3 items=["Channel 1", "Channel 2", "Channel 3", "Channel 4", "Math 1", "Math 2", "Math 3", "Math 4", "Reference 1", "Reference 2", "Reference 3", "Reference 4"] ("Channel")
              n227 = call "Channel_Active_Request.vi"("Command"="SEL:CH4?", "VISA resource name"=w433) -> ("error out"=w434:errorcluster, "Active?"=w432:bool, "VISA resource name out"=w436:refnum<visa-resource-name>)  [unwired: 6 in, 1 out]
              n228 = case shown="True" w432 {
                selector: w432 -> [w438 w452]
                tunnel: w436 -> [w442 w454]
                tunnel: [w440 w456] -> w435
                tunnel: w434 -> [w439 w455]
                tunnel: w431 -> [w443 w451]
                frame False {
                  n229 = local read "Ch 4"() -> (w441:bool)
                  n230 = case shown="True" w441 {
                    tunnel: w443 -> [_ w447]
                    tunnel: w442 -> [_ w446]
                    tunnel: [w444 w450] -> w440
                    tunnel: w439 -> [w444 w449]
                    tunnel: w438 -> [_ w448]
                    frame False {
                    }
                    frame True {
                      n231 = call "DPO_7K_Enable_Channel.vi"("Error In"=w449, "Activate?"=w448, "Channel"=w447, "VISA resource name in"=w446) -> ("Error Out"=w450:errorcluster, "State_Channel"=w445:bool)  [unwired: 5 in, 1 out]
                      n232 = local write "Ch 4"(w445) -> ()
                      n233 = local write "S4"(w445) -> ()
                    }
                  }
                }
                frame True {
                  n234 = local read "Ch 4"() -> (w453:bool)
                  n235 = case shown="False" w453 {
                    tunnel: w454 -> [w462 _]
                    tunnel: [w461 w463] -> w456
                    tunnel: w455 -> [w460 w463]
                    tunnel: w452 -> [w459 _]
                    tunnel: w451 -> [w458 _]
                    frame False {
                      n236 = call "DPO_7K_Enable_Channel.vi"("Error In"=w460, "Activate?"=w459, "Channel"=w458, "VISA resource name in"=w462) -> ("Error Out"=w461:errorcluster, "State_Channel"=w457:bool)  [unwired: 5 in, 1 out]
                      n237 = local write "Ch 4"(w457) -> ()
                      n238 = local write "S4"(w457) -> ()
                    }
                    frame True {
                    }
                  }
                }
              }
            }
          }
        }
        n239 = local write "Synch Variable"(w323) -> ()
      }
      event "Play Button": Value Change {
        w465 = u16 0 items=["Run", "Stop"] ("Action")
        n240 = event-data() -> ()  [unwired: 1 in, 6 out]
        n241 = local read "Set Oscilloscope Mode"() -> (w464:u16)
        n242 = local write "Running?"(TRUE ("Running?")) -> ()
        n243 = call "DPO_7K_Acquisition Mode.vi"("Mode"=w464, "Action"=w465, "VISA resource name in"=w467) -> ("Error Out"=w466:errorcluster)  [unwired: 7 in, 1 out]
      }
      event "Pause Button": Value Change {
        w470 = u16 1 items=["Run", "Stop"] ("Action")
        n244 = event-data() -> ()  [unwired: 1 in, 6 out]
        n245 = local read "Set Oscilloscope Mode"() -> (w469:u16)
        n246 = call "DPO_7K_Acquisition Mode.vi"("Mode"=w469, "Action"=w470, "VISA resource name in"=w472) -> ("Error Out"=w471:errorcluster)  [unwired: 7 in, 1 out]
        n247 = local write "Running?"(FALSE ("Running?")) -> ()
      }
    }
    n248 = case shown="Error .." w129 {
      selector: w129 -> [_ w132]
      frame No Error {
        # "handles errors"
      }
      frame Error {
        # "handles errors"
        n249 = call <vilib>:"Simple Error Handler.vi"("error in (no error)"=w132) -> ()  [unwired: 4 in, 5 out]
      }
    }
  }
  n250 = while {
    shift-right: [w494] -> w11
    shift-left: w13 -> [w497]
    tunnel: w12 -> [w495]
    tunnel: [w496] -> w10
    tunnel: w7 -> [w486]
    stop <- w492 stop-if-true
    # "speed"
    # "Acquires  Signals on the Channels"
    n251 = for {
      N: 4 -> [_]
      shift-right: [w514] -> w483
      shift-left: u16[] [] ("array") -> [w515]
      tunnel: w486 -> [w513]
      tunnel: [w512] -> w487
      tunnel: [w511] -> w488
      i -> [w516]
      # "Create an array of active channels"
      n252 = case shown="2" w516 {
        tunnel: w515 -> [w521 w557 w594 w629]
        tunnel: [w520 w556 w593 w628] -> w514
        tunnel: w513 -> [w519 w554 w590 w627]
        tunnel: [w518 w555 w592 w626] -> w512
        tunnel: [w517 w553 w591 w625] -> w511
        frame 0, Default {
          w522 = u16 0 items=["Channel1", "Channel2", "Channel3", "Channel4", "Math1", "Math2", "Math3", "Math3", "Reference1", "Reference2", "Reference3", "Reference4"] ("Channel (0:Channel1)")
          n253 = local read "Ch 1"() -> (w523:bool)
          n254 = case shown="True" w523 {
            selector: w523 -> [w528 w539]
            tunnel: w522 -> [w529 w543]
            tunnel: w521 -> [w530 w545]
            tunnel: [w530 w544] -> w520
            tunnel: w519 -> [w527 w542]
            tunnel: [w526 w541] -> w518
            tunnel: [w525 w540] -> w517
            frame False {
              n255 = local read "S1"() -> (w524:bool)
              n256 = case shown="True" w524 {
                tunnel: w529 -> [_ w537]
                tunnel: w528 -> [_ w536]
                tunnel: w527 -> [w531 w535]
                tunnel: [_ w534] -> w526
                tunnel: [w531 w533] -> w525
                frame False {
                }
                frame True {
                  n257 = call "DPO_7K_Enable_Channel.vi"("Activate?"=w536, "Channel"=w537, "VISA resource name in"=w535) -> ("Error Out"=w534:errorcluster, "State_Channel"=w532:bool, "VISA resource name out"=w533:refnum<visa-resource-name>)  [unwired: 6 in]
                  n258 = local write "S1"(w532) -> ()
                }
              }
            }
            frame True {
              n259 = local read "S1"() -> (w538:bool)
              n260 = case shown="True" w538 {
                tunnel: w543 -> [w551 _]
                tunnel: w542 -> [w550 w552]
                tunnel: [w549 _] -> w541
                tunnel: [w548 w552] -> w540
                tunnel: w539 -> [w547 _]
                frame False {
                  n261 = call "DPO_7K_Enable_Channel.vi"("Activate?"=w547, "Channel"=w551, "VISA resource name in"=w550) -> ("Error Out"=w549:errorcluster, "State_Channel"=w546:bool, "VISA resource name out"=w548:refnum<visa-resource-name>)  [unwired: 6 in]
                  n262 = local write "S1"(w546) -> ()
                }
                frame True {
                }
              }
              n263 = Insert Into Array(array=w545, new element=w543) -> (w544:u16[])  [unwired: 1 in]
            }
          }
        }
        frame 1 {
          w558 = u16 1 items=["Channel1", "Channel2", "Channel3", "Channel4", "Math1", "Math2", "Math3", "Math3", "Reference1", "Reference2", "Reference3", "Reference4"] ("Channel (0:Channel1)")
          n264 = local read "Ch 2"() -> (w559:bool)
          n265 = case shown="False" w559 {
            selector: w559 -> [w564 w578]
            tunnel: w558 -> [w565 w579]
            tunnel: w557 -> [w566 w580]
            tunnel: [w566 w581] -> w556
            tunnel: [w563 w577] -> w555
            tunnel: w554 -> [w562 w576]
            tunnel: [w561 w575] -> w553
            frame False {
              n266 = local read "S2"() -> (w560:bool)
              n267 = case shown="False" w560 {
                tunnel: w565 -> [_ w573]
                tunnel: w564 -> [_ w572]
                tunnel: [_ w571] -> w563
                tunnel: w562 -> [w567 w570]
                tunnel: [w567 w569] -> w561
                frame False {
                }
                frame True {
                  n268 = call "DPO_7K_Enable_Channel.vi"("Activate?"=w572, "Channel"=w573, "VISA resource name in"=w570) -> ("Error Out"=w571:errorcluster, "State_Channel"=w568:bool, "VISA resource name out"=w569:refnum<visa-resource-name>)  [unwired: 6 in]
                  n269 = local write "S2"(w568) -> ()
                }
              }
            }
            frame True {
              n270 = local read "S2"() -> (w574:bool)
              n271 = case shown="True" w574 {
                tunnel: w579 -> [w587 _]
                tunnel: w578 -> [w586 _]
                tunnel: [w585 _] -> w577
                tunnel: w576 -> [w584 w588]
                tunnel: [w583 w588] -> w575
                frame False {
                  n272 = call "DPO_7K_Enable_Channel.vi"("Activate?"=w586, "Channel"=w587, "VISA resource name in"=w584) -> ("Error Out"=w585:errorcluster, "State_Channel"=w582:bool, "VISA resource name out"=w583:refnum<visa-resource-name>)  [unwired: 6 in]
                  n273 = local write "S2"(w582) -> ()
                }
                frame True {
                }
              }
              n274 = Insert Into Array(array=w580, new element=w579) -> (w581:u16[])  [unwired: 1 in]
            }
          }
        }
        frame 2 {
          w595 = u16 2 items=["Channel1", "Channel2", "Channel3", "Channel4", "Math1", "Math2", "Math3", "Math3", "Reference1", "Reference2", "Reference3", "Reference4"] ("Channel (0:Channel1)")
          n275 = local read "Ch 3"() -> (w589:bool)
          n276 = case shown="True" w589 {
            selector: w589 -> [w600 w614]
            tunnel: w595 -> [w601 w615]
            tunnel: w594 -> [w602 w617]
            tunnel: [w602 w616] -> w593
            tunnel: w590 -> [w599 w613]
            tunnel: [w598 w612] -> w592
            tunnel: [w597 w611] -> w591
            frame False {
              n277 = local read "S3"() -> (w596:bool)
              n278 = case shown="False" w596 {
                tunnel: w601 -> [_ w609]
                tunnel: w600 -> [_ w608]
                tunnel: w599 -> [w603 w607]
                tunnel: [_ w606] -> w598
                tunnel: [w603 w605] -> w597
                frame False {
                }
                frame True {
                  n279 = call "DPO_7K_Enable_Channel.vi"("Activate?"=w608, "Channel"=w609, "VISA resource name in"=w607) -> ("Error Out"=w606:errorcluster, "State_Channel"=w604:bool, "VISA resource name out"=w605:refnum<visa-resource-name>)  [unwired: 6 in]
                  n280 = local write "S3"(w604) -> ()
                }
              }
            }
            frame True {
              n281 = local read "S3"() -> (w610:bool)
              n282 = case shown="False" w610 {
                tunnel: w615 -> [w623 _]
                tunnel: w614 -> [w622 _]
                tunnel: w613 -> [w621 w624]
                tunnel: [w620 _] -> w612
                tunnel: [w619 w624] -> w611
                frame False {
                  n283 = call "DPO_7K_Enable_Channel.vi"("Activate?"=w622, "Channel"=w623, "VISA resource name in"=w621) -> ("Error Out"=w620:errorcluster, "State_Channel"=w618:bool, "VISA resource name out"=w619:refnum<visa-resource-name>)  [unwired: 6 in]
                  n284 = local write "S3"(w618) -> ()
                }
                frame True {
                }
              }
              n285 = Insert Into Array(array=w617, new element=w615) -> (w616:u16[])  [unwired: 1 in]
            }
          }
        }
        frame 3 {
          w630 = u16 3 items=["Channel1", "Channel2", "Channel3", "Channel4", "Math1", "Math2", "Math3", "Math3", "Reference1", "Reference2", "Reference3", "Reference4"] ("Channel (0:Channel1)")
          n286 = local read "Ch 4"() -> (w631:bool)
          n287 = case shown="True" w631 {
            selector: w631 -> [w636 w650]
            tunnel: w630 -> [w637 w651]
            tunnel: w629 -> [w638 w653]
            tunnel: [w638 w652] -> w628
            tunnel: w627 -> [w635 w649]
            tunnel: [w634 w648] -> w626
            tunnel: [w633 w647] -> w625
            frame False {
              n288 = local read "S4"() -> (w632:bool)
              n289 = case shown="False" w632 {
                tunnel: w637 -> [_ w645]
                tunnel: w636 -> [_ w644]
                tunnel: w635 -> [w639 w643]
                tunnel: [_ w642] -> w634
                tunnel: [w639 w641] -> w633
                frame False {
                }
                frame True {
                  n290 = call "DPO_7K_Enable_Channel.vi"("Activate?"=w644, "Channel"=w645, "VISA resource name in"=w643) -> ("Error Out"=w642:errorcluster, "State_Channel"=w640:bool, "VISA resource name out"=w641:refnum<visa-resource-name>)  [unwired: 6 in]
                  n291 = local write "S4"(w640) -> ()
                }
              }
            }
            frame True {
              n292 = local read "S4"() -> (w646:bool)
              n293 = case shown="True" w646 {
                tunnel: w651 -> [w659 _]
                tunnel: w650 -> [w658 _]
                tunnel: w649 -> [w657 w660]
                tunnel: [w656 _] -> w648
                tunnel: [w655 w660] -> w647
                frame False {
                  n294 = call "DPO_7K_Enable_Channel.vi"("Activate?"=w658, "Channel"=w659, "VISA resource name in"=w657) -> ("Error Out"=w656:errorcluster, "State_Channel"=w654:bool, "VISA resource name out"=w655:refnum<visa-resource-name>)  [unwired: 6 in]
                  n295 = local write "S4"(w654) -> ()
                }
                frame True {
                }
              }
              n296 = Insert Into Array(array=w653, new element=w651) -> (w652:u16[])  [unwired: 1 in]
            }
          }
        }
      }
    }
    "Active_Channels" <- w483
    n297 = local read "Synch Variable"() -> (w477:bool)
    n298 = case shown="True" w477 {
      tunnel: w488 -> [w505 w510]
      tunnel: w487 -> [w504 w508]
      tunnel: [w503 w510] -> w485
      tunnel: [w499 w507] -> w484
      tunnel: w483 -> [w502 w509]
      tunnel: [w501 w509] -> w478
      tunnel: [w500 w508] -> w476
      tunnel: [w499 w507] -> w475
      tunnel: [TRUE FALSE] -> w474
      frame False {
        # "waveforms"
        n299 = call "DPO_7K_Read Multiple Waveforms.vi"("error in (no error)"=w504, "Channels"=w502, "VISA resource name"=w505) -> ("error out"=w500:errorcluster, "ChannelsArray"=w501:u16[], "Waveform Data"=w499:waveform(dbl)[], "VISA resource name out"=w503:refnum<visa-resource-name>)  [unwired: 5 in]
        n300 = call <vilib>:"Simple Error Handler.vi"("error in (no error)"=w500) -> ()  [unwired: 4 in, 5 out]
      }
      frame True {
        w507 = waveform(dbl)[] [] ("Waveform Data")
      }
    }
    "Tektronix 7000 Oscilloscope" <- w475
    n301 = local read "Save Variable"() -> (w481:bool)
    n302 = local read "Go!"() -> (w480:bool)
    n303 = Not(x=w480) -> (.not. x?=w479:bool)
    n304 = And(x=w481, y=w479) -> (x .and. y?=w482:bool)
    n305 = case shown="True" w482 {
      tunnel: w497 -> [w662 w676]
      tunnel: [w663 w675] -> w496
      tunnel: w495 -> [w663 w674]
      tunnel: [w662 w673] -> w494
      tunnel: w484 -> [_ w671]
      tunnel: w478 -> [_ w664]
      tunnel: w485 -> [_ w670]
      tunnel: w476 -> [_ w668]
      tunnel: w474 -> [_ w666]
      frame False {
        # "Queue the entire waveform of the graph once pressed the save button"
        n306 = local write "Display Message"("Oscilloscope" ("Message")) -> ()
      }
      frame True {
        # "data"
        # "settings"
        # "Queue the entire waveform of the graph once pressed the save button"
        n307 = call "Parameters_Request.vi"("error in (no error)"=w668, "Active Channels"=w664, "VISA resource name"=w670) -> ("error out"=w667:errorcluster, "Parameters(array)"=w669:string[])  [unwired: 6 in, 1 out]
        n308 = Bundle("Parameters(array)"=w669, "Waveform Data"=w671, "array"=w664, w666) -> (w665:T2)  [unwired: 1 in]
        n309 = case shown="No Error" w667 {
          selector: w667 -> [_ w681]
          tunnel: w665 -> [w678 w680]
          frame No Error {
            n310 = Unbundle(w678) -> (w677:bool)  [unwired: 3 out]
            n311 = local write "Go!"(w677) -> ()
          }
          frame Error {
            n312 = Unbundle(w680) -> (w679:bool)  [unwired: 3 out]
            n313 = local write "Go!"(w679) -> ()
            n314 = call <vilib>:"Simple Error Handler.vi"("error in (no error)"=w681) -> ()  [unwired: 4 in, 5 out]
          }
        }
        n315 = local write "Display Message"("Saving Data" ("Message")) -> ()
        n316 = Enqueue Element(queue=w674, element=w665, error in (no error)=w676) -> (queue out=w675:refnum<queue>, error out=w673:errorcluster)  [unwired: 1 in, 1 out]
      }
    }
    n317 = local read "End Variable"() -> (w489:bool)
    n318 = Or(x=w494, y=w489) -> (x .or. y?=w492:bool)
    n319 = Wait (ms)(milliseconds to wait=u32 200) -> ()  [unwired: 1 out]
  }
  n320 = Release Queue(queue=w10, error in (no error)=w11) -> (error out=w9:errorcluster)  [unwired: 1 in, 2 out]
  n321 = call <vilib>:"Simple Error Handler.vi"("error in (no error)"=w9) -> ("error?"=w8:bool)  [unwired: 4 in, 4 out]
  n322 = Stop(stop? (T)=w8) -> ()
